vi "WaitError.vi"(2 "error in (no error)":errorcluster, 3 "Wait time (ms)":dbl) -> (0 "error out":errorcluster)   [LabVIEW 2011]
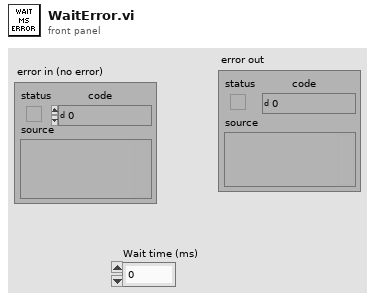
[diagram p1: front panel]
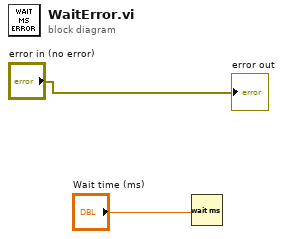
[diagram p0: block diagram]
diagram:
  n1 = Wait (ms)(milliseconds to wait="Wait time (ms)") -> ()  [unwired: 1 out]
  "error out" <- "error in (no error)"
